vi "ins2pac.vi"(1 "BODY":i8[](array[numeric]), 2 "chn num":u16, 3 "SEQUENCE":u32, 4 "TYPE":T1(ring)) -> (0 "PACKET":string)   [LabVIEW 2016]
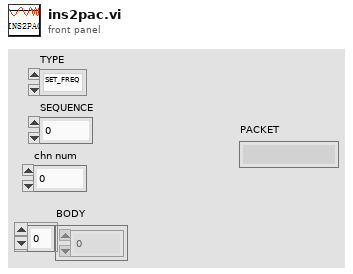
[diagram p1: front panel]
types:
  T1 = enum8{"SET_FREQ", "SET_VOLT", "SET_CHANNEL_VOLT", "SET_PHASE", "START_HEAT", "STOP_HEAT", "CHANNEL_CTRL_SINGLE", "CHANNEL_CTRL_ALL", "READ_VOLT_SET", "READ_VOLT_SET_RSP", "READ_CURRENT_VOLT", "READ_CURRENT_VOLT_RSP", "READ_PHASE", "READ_PHASE_RSP", "READ_HEATTIME_LEFT", "READ_HEATTIME_LEFT_RSP", "EXEC_RSP"}
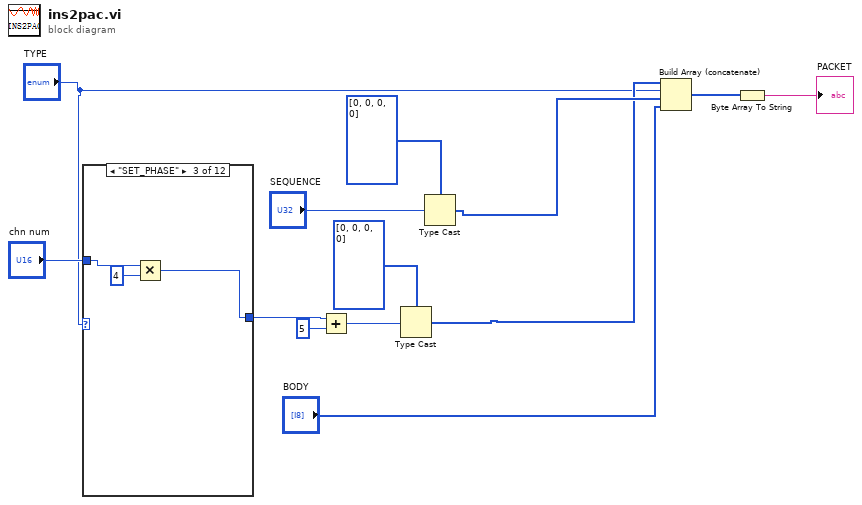
[diagram p0: block diagram]
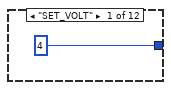
[diagram p2: hidden frame]
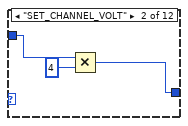
[diagram p3: hidden frame]
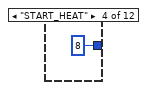
[diagram p4: hidden frame]
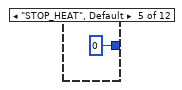
[diagram p5: hidden frame]
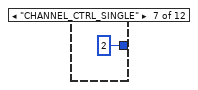
[diagram p7: hidden frame]
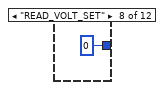
[diagram p8: hidden frame]
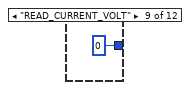
[diagram p9: hidden frame]
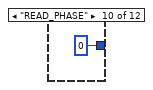
[diagram p10: hidden frame]
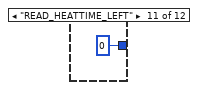
[diagram p11: hidden frame]
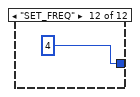
[diagram p12: hidden frame]
diagram:
  n1 = case shown="\"SET_PHASE\"" "TYPE" {
    tunnel: "chn num" -> [_ w17 w20 _ _ w23 _ _ _ _ _ _]
    tunnel: [4 w15 w18 8 ("chn num") 0 ("chn num") w23 2 ("chn num") 0 ("chn num") 0 ("chn num") 0 ("chn num") 0 ("chn num") 4] -> w6
    frame "SET_VOLT" {
    }
    frame "SET_CHANNEL_VOLT" {
      n2 = Multiply(x=w17, y=u16 4) -> (x*y=w15:u16)
    }
    frame "SET_PHASE" {
      n3 = Multiply(x=w20, y=u16 4) -> (x*y=w18:u16)
    }
    frame "START_HEAT" {
    }
    frame "STOP_HEAT", Default {
    }
    frame "CHANNEL_CTRL_ALL" {
    }
    frame "CHANNEL_CTRL_SINGLE" {
    }
    frame "READ_VOLT_SET" {
    }
    frame "READ_CURRENT_VOLT" {
    }
    frame "READ_PHASE" {
    }
    frame "READ_HEATTIME_LEFT" {
    }
    frame "SET_FREQ" {
    }
  }
  n4 = Add(x=w6, y=5) -> (x+y=w4:i32)
  n5 = Type Cast(type=u8[] [0, 0, 0, 0], x=w4) -> (*(type *) &x=w2:u8[])
  n6 = Type Cast(type=u8[] [0, 0, 0, 0], x="SEQUENCE") -> (*(type *) &x=w3:u8[])
  n7 = Build Array (concatenate)(w2, "TYPE", w3, "BODY") -> (w9:u8[])
  n8 = Byte Array To String(unsigned byte array=w9) -> (string=→"PACKET":string)
